vi "test TCX read (installed 71).vi"() -> ()   [LabVIEW 2011] (continued)
xmlns=\"http://www.garmin.com/xmlschemas/ActivityExtension/v2\"><Watts>67</Watts></TPX></Extensions></Trackpoint><Trackpoint><Time>2008-03-03T23:25:10Z</Time><Position><LatitudeDegrees>35.887956</LatitudeDegrees><LongitudeDegrees>-78.948106</LongitudeDegrees></Position><AltitudeMeters>75.120</AltitudeMeters><DistanceMeters>21918.861</DistanceMeters><Cadence>88</Cadence><Extensions><TPX xmlns=\"http://www.garmin.com/xmlschemas/ActivityExtension/v2\"><Watts>54</Watts></TPX></Extensions></Trackpoint><Trackpoint><Time>2008-03-03T23:25:11Z</Time><Position><LatitudeDegrees>35.888009</LatitudeDegrees><LongitudeDegrees>-78.948257</LongitudeDegrees></Position><AltitudeMeters>74.640</AltitudeMeters><DistanceMeters>21933.953</DistanceMeters><Cadence>89</Cadence><Extensions><TPX xmlns=\"http://www.garmin.com/xmlschemas/ActivityExtension/v2\"><Watts>47</Watts></TPX></Extensions></Trackpoint><Trackpoint><Time>2008-03-03T23:25:12Z</Time><Position><LatitudeDegrees>35.888052</LatitudeDegrees><LongitudeDegrees>-78.948414</LongitudeDegrees></Position><AltitudeMeters>72.717</AltitudeMeters><DistanceMeters>21948.695</DistanceMeters><Cadence>90</Cadence><Extensions><TPX xmlns=\"http://www.garmin.com/xmlschemas/ActivityExtension/v2\"><Watts>43</Watts></TPX></Extensions></Trackpoint><Trackpoint><Time>2008-03-03T23:25:13Z</Time><Position><LatitudeDegrees>35.888082</LatitudeDegrees><LongitudeDegrees>-78.948575</LongitudeDegrees></Position><AltitudeMeters>72.236</AltitudeMeters><DistanceMeters>21963.564</DistanceMeters><Cadence>89</Cadence><Extensions><TPX xmlns=\"http://www.garmin.com/xmlschemas/ActivityExtension/v2\"><Watts>44</Watts></TPX></Extensions></Trackpoint><Trackpoint><Time>2008-03-03T23:25:14Z</Time><Position><LatitudeDegrees>35.888095</LatitudeDegrees><LongitudeDegrees>-78.948737</LongitudeDegrees></Position><AltitudeMeters>72.236</AltitudeMeters><DistanceMeters>21978.184</DistanceMeters><Cadence>87</Cadence><Extensions><TPX xmlns=\"http://www.garmin.com/xmlschemas/ActivityExtension/v2\"><Watts>41</Watts></TPX></Extensions></Trackpoint><Trackpoint><Time>2008-03-03T23:25:15Z</Time><Position><LatitudeDegrees>35.888094</LatitudeDegrees><LongitudeDegrees>-78.948896</LongitudeDegrees></Position><AltitudeMeters>72.236</AltitudeMeters><DistanceMeters>21992.566</DistanceMeters><Cadence>87</Cadence><Extensions><TPX xmlns=\"http://www.garmin.com/xmlschemas/ActivityExtension/v2\"><Watts>41</Watts></TPX></Extensions></Trackpoint><Trackpoint><Time>2008-03-03T23:25:16Z</Time><Position><LatitudeDegrees>35.888082</LatitudeDegrees><LongitudeDegrees>-78.949051</LongitudeDegrees></Position><AltitudeMeters>71.755</AltitudeMeters><DistanceMeters>22006.510</DistanceMeters><Cadence>0</Cadence></Trackpoint><Trackpoint><Time>2008-03-03T23:25:17Z</Time><Position><LatitudeDegrees>35.888058</LatitudeDegrees><LongitudeDegrees>-78.949199</LongitudeDegrees></Position><AltitudeMeters>71.275</AltitudeMeters><DistanceMeters>22020.152</DistanceMeters><Cadence>0</Cadence></Trackpoint><Trackpoint><Time>2008-03-03T23:25:18Z</Time><Position><LatitudeDegrees>35.888029</LatitudeDegrees><LongitudeDegrees>-78.949342</LongitudeDegrees></Position><AltitudeMeters>71.275</AltitudeMeters><DistanceMeters>22033.473</DistanceMeters><Cadence>17</Cadence></Trackpoint><Trackpoint><Time>2008-03-03T23:25:19Z</Time><Position><LatitudeDegrees>35.888005</LatitudeDegrees><LongitudeDegrees>-78.949482</LongitudeDegrees></Position><AltitudeMeters>71.275</AltitudeMeters><DistanceMeters>22046.338</DistanceMeters><Cadence>33</Cadence></Trackpoint><Trackpoint><Time>2008-03-03T23:25:20Z</Time><Position><LatitudeDegrees>35.888007</LatitudeDegrees><LongitudeDegrees>-78.949623</LongitudeDegrees></Position><AltitudeMeters>70.794</AltitudeMeters><DistanceMeters>22058.844</DistanceMeters><Cadence>33</Cadence></Trackpoint><Trackpoint><Time>2008-03-03T23:25:21Z</Time><Position><LatitudeDegrees>35.888061</LatitudeDegrees><LongitudeDegrees>-78.949736</LongitudeDegrees></Position><AltitudeMeters>70.794</AltitudeMeters><DistanceMeters>22070.695</DistanceMeters><Cadence>0</Cadence></Trackpoint><Trackpoint><Time>2008-03-03T23:25:22Z</Time><Position><LatitudeDegrees>35.888146</LatitudeDegrees><LongitudeDegrees>-78.949802</LongitudeDegrees></Position><AltitudeMeters>70.794</AltitudeMeters><DistanceMeters>22081.836</DistanceMeters><Cadence>89</Cadence><Extensions><TPX xmlns=\"http://www.garmin.com/xmlschemas/ActivityExtension/v2\"><Watts>68</Watts></TPX></Extensions></Trackpoint><Trackpoint><Time>2008-03-03T23:25:23Z</Time><Position><LatitudeDegrees>35.888236</LatitudeDegrees><LongitudeDegrees>-78.949853</LongitudeDegrees></Position><AltitudeMeters>70.794</AltitudeMeters><DistanceMeters>22092.775</DistanceMeters><Cadence>89</Cadence><Extensions><TPX xmlns=\"http://www.garmin.com/xmlschemas/ActivityExtension/v2\"><Watts>73</Watts></TPX></Extensions></Trackpoint><Trackpoint><Time>2008-03-03T23:25:24Z</Time><Position><LatitudeDegrees>35.888330</LatitudeDegrees><LongitudeDegrees>-78.949892</LongitudeDegrees></Position><AltitudeMeters>70.794</AltitudeMeters><DistanceMeters>22103.824</DistanceMeters><Cadence>80</Cadence><Extensions><TPX xmlns=\"http://www.garmin.com/xmlschemas/ActivityExtension/v2\"><Watts>113</Watts></TPX></Extensions></Trackpoint><Trackpoint><Time>2008-03-03T23:25:25Z</Time><Position><LatitudeDegrees>35.888423</LatitudeDegrees><LongitudeDegrees>-78.949920</LongitudeDegrees></Position><AltitudeMeters>70.794</AltitudeMeters><DistanceMeters>22114.348</DistanceMeters><Cadence>80</Cadence><Extensions><TPX xmlns=\"http://www.garmin.com/xmlschemas/ActivityExtension/v2\"><Watts>112</Watts></TPX></Extensions></Trackpoint><Trackpoint><Time>2008-03-03T23:25:26Z</Time><Position><LatitudeDegrees>35.888512</LatitudeDegrees><LongitudeDegrees>-78.949941</LongitudeDegrees></Position><AltitudeMeters>70.794</AltitudeMeters><DistanceMeters>22124.379</DistanceMeters><Cadence>82</Cadence><Extensions><TPX xmlns=\"http://www.garmin.com/xmlschemas/ActivityExtension/v2\"><Watts>127</Watts></TPX></Extensions></Trackpoint><Trackpoint><Time>2008-03-03T23:25:27Z</Time><Position><LatitudeDegrees>35.888597</LatitudeDegrees><LongitudeDegrees>-78.949963</LongitudeDegrees></Position><AltitudeMeters>70.313</AltitudeMeters><DistanceMeters>22134.072</DistanceMeters><Cadence>78</Cadence><Extensions><TPX xmlns=\"http://www.garmin.com/xmlschemas/ActivityExtension/v2\"><Watts>137</Watts></TPX></Extensions></Trackpoint><Trackpoint><Time>2008-03-03T23:25:28Z</Time><Position><LatitudeDegrees>35.888682</LatitudeDegrees><LongitudeDegrees>-78.949991</LongitudeDegrees></Position><AltitudeMeters>70.794</AltitudeMeters><DistanceMeters>22143.781</DistanceMeters><Cadence>78</Cadence><Extensions><TPX xmlns=\"http://www.garmin.com/xmlschemas/ActivityExtension/v2\"><Watts>234</Watts></TPX></Extensions></Trackpoint><Trackpoint><Time>2008-03-03T23:25:29Z</Time><Position><LatitudeDegrees>35.888765</LatitudeDegrees><LongitudeDegrees>-78.950025</LongitudeDegrees></Position><AltitudeMeters>70.794</AltitudeMeters><DistanceMeters>22153.506</DistanceMeters><Cadence>78</Cadence><Extensions><TPX xmlns=\"http://www.garmin.com/xmlschemas/ActivityExtension/v2\"><Watts>358</Watts></TPX></Extensions></Trackpoint><Trackpoint><Time>2008-03-03T23:25:30Z</Time><Position><LatitudeDegrees>35.888845</LatitudeDegrees><LongitudeDegrees>-78.950066</LongitudeDegrees></Position><AltitudeMeters>71.275</AltitudeMeters><DistanceMeters>22163.023</DistanceMeters><Cadence>78</Cadence><Extensions><TPX xmlns=\"http://www.garmin.com/xmlschemas/ActivityExtension/v2\"><Watts>358</Watts></TPX></Extensions></Trackpoint><Trackpoint><Time>2008-03-03T23:25:31Z</Time><Position><LatitudeDegrees>35.888920</LatitudeDegrees><LongitudeDegrees>-78.950108</LongitudeDegrees></Position><AltitudeMeters>71.755</AltitudeMeters><DistanceMeters>22172.158</DistanceMeters><Cadence>73</Cadence><Extensions><TPX xmlns=\"http://www.garmin.com/xmlschemas/ActivityExtension/v2\"><Watts>561</Watts></TPX></Extensions></Trackpoint><Trackpoint><Time>2008-03-03T23:25:32Z</Time><Position><LatitudeDegrees>35.888993</LatitudeDegrees><LongitudeDegrees>-78.950147</LongitudeDegrees></Position><AltitudeMeters>72.717</AltitudeMeters><DistanceMeters>22181.043</DistanceMeters><Cadence>71</Cadence><Extensions><TPX xmlns=\"http://www.garmin.com/xmlschemas/ActivityExtension/v2\"><Watts>610</Watts></TPX></Extensions></Trackpoint><Trackpoint><Time>2008-03-03T23:25:33Z</Time><Position><LatitudeDegrees>35.889063</LatitudeDegrees><LongitudeDegrees>-78.950189</LongitudeDegrees></Position><AltitudeMeters>73.198</AltitudeMeters><DistanceMeters>22189.660</DistanceMeters><Cadence>71</Cadence><Extensions><TPX xmlns=\"http://www.garmin.com/xmlschemas/ActivityExtension/v2\"><Watts>609</Watts></TPX></Extensions></Trackpoint><Trackpoint><Time>2008-03-03T23:25:34Z</Time><Position><LatitudeDegrees>35.889129</LatitudeDegrees><LongitudeDegrees>-78.950236</LongitudeDegrees></Position><AltitudeMeters>74.159</AltitudeMeters><DistanceMeters>22198.082</DistanceMeters><Cadence>68</Cadence><Extensions><TPX xmlns=\"http://www.garmin.com/xmlschemas/ActivityExtension/v2\"><Watts>594</Watts></TPX></Extensions></Trackpoint><Trackpoint><Time>2008-03-03T23:25:35Z</Time><Position><LatitudeDegrees>35.889194</LatitudeDegrees><LongitudeDegrees>-78.950285</LongitudeDegrees></Position><AltitudeMeters>74.640</AltitudeMeters><DistanceMeters>22206.525</DistanceMeters><Cadence>67</Cadence><Extensions><TPX xmlns=\"http://www.garmin.com/xmlschemas/ActivityExtension/v2\"><Watts>574</Watts></TPX></Extensions></Trackpoint><Trackpoint><Time>2008-03-03T23:25:36Z</Time><Position><LatitudeDegrees>35.889252</LatitudeDegrees><LongitudeDegrees>-78.950341</LongitudeDegrees></Position><AltitudeMeters>74.640</AltitudeMeters><DistanceMeters>22214.654</DistanceMeters><Cadence>67</Cadence><Extensions><TPX xmlns=\"http://www.garmin.com/xmlschemas/ActivityExtension/v2\"><Watts>549</Watts></TPX></Extensions></Trackpoint><Trackpoint><Time>2008-03-03T23:25:37Z</Time><Position><LatitudeDegrees>35.889306</LatitudeDegrees><LongitudeDegrees>-78.950404</LongitudeDegrees></Position><AltitudeMeters>75.120</AltitudeMeters><DistanceMeters>22222.992</DistanceMeters><Cadence>67</Cadence><Extensions><TPX xmlns=\"http://www.garmin.com/xmlschemas/ActivityExtension/v2\"><Watts>534</Watts></TPX></Extensions></Trackpoint><Trackpoint><Time>2008-03-03T23:25:38Z</Time><Position><LatitudeDegrees>35.889357</LatitudeDegrees><LongitudeDegrees>-78.950472</LongitudeDegrees></Position><AltitudeMeters>75.601</AltitudeMeters><DistanceMeters>22231.277</DistanceMeters><Cadence>67</Cadence><Extensions><TPX xmlns=\"http://www.garmin.com/xmlschemas/ActivityExtension/v2\"><Watts>523</Watts></TPX></Extensions></Trackpoint><Trackpoint><Time>2008-03-03T23:25:39Z</Time><Position><LatitudeDegrees>35.889403</LatitudeDegrees><LongitudeDegrees>-78.950544</LongitudeDegrees></Position><AltitudeMeters>75.601</AltitudeMeters><DistanceMeters>22239.598</DistanceMeters><Cadence>69</Cadence><Extensions><TPX xmlns=\"http://www.garmin.com/xmlschemas/ActivityExtension/v2\"><Watts>356</Watts></TPX></Extensions></Trackpoint><Trackpoint><Time>2008-03-03T23:25:40Z</Time><Position><LatitudeDegrees>35.889447</LatitudeDegrees><LongitudeDegrees>-78.950625</LongitudeDegrees></Position><AltitudeMeters>76.562</AltitudeMeters><DistanceMeters>22248.361</DistanceMeters><Cadence>69</Cadence><Extensions><TPX xmlns=\"http://www.garmin.com/xmlschemas/ActivityExtension/v2\"><Watts>353</Watts></TPX></Extensions></Trackpoint><Trackpoint><Time>2008-03-03T23:25:41Z</Time><Position><LatitudeDegrees>35.889484</LatitudeDegrees><LongitudeDegrees>-78.950711</LongitudeDegrees></Position><AltitudeMeters>76.081</AltitudeMeters><DistanceMeters>22257.133</DistanceMeters><Cadence>71</Cadence><Extensions><TPX xmlns=\"http://www.garmin.com/xmlschemas/ActivityExtension/v2\"><Watts>275</Watts></TPX></Extensions></Trackpoint><Trackpoint><Time>2008-03-03T23:25:42Z</Time><Position><LatitudeDegrees>35.889518</LatitudeDegrees><LongitudeDegrees>-78.950802</LongitudeDegrees></Position><AltitudeMeters>75.601</AltitudeMeters><DistanceMeters>22266.189</DistanceMeters><Cadence>71</Cadence><Extensions><TPX xmlns=\"http://www.garmin.com/xmlschemas/ActivityExtension/v2\"><Watts>270</Watts></TPX></Extensions></Trackpoint><Trackpoint><Time>2008-03-03T23:25:43Z</Time><Position><LatitudeDegrees>35.889549</LatitudeDegrees><LongitudeDegrees>-78.950897</LongitudeDegrees></Position><AltitudeMeters>76.081</AltitudeMeters><DistanceMeters>22275.441</DistanceMeters><Cadence>77</Cadence><Extensions><TPX xmlns=\"http://www.garmin.com/xmlschemas/ActivityExtension/v2\"><Watts>84</Watts></TPX></Extensions></Trackpoint><Trackpoint><Time>2008-03-03T23:25:44Z</Time><Position><LatitudeDegrees>35.889575</LatitudeDegrees><LongitudeDegrees>-78.950998</LongitudeDegrees></Position><AltitudeMeters>75.601</AltitudeMeters><DistanceMeters>22285.012</DistanceMeters><Cadence>79</Cadence><Extensions><TPX xmlns=\"http://www.garmin.com/xmlschemas/ActivityExtension/v2\"><Watts>51</Watts></TPX></Extensions></Trackpoint><Trackpoint><Time>2008-03-03T23:25:45Z</Time><Position><LatitudeDegrees>35.889595</LatitudeDegrees><LongitudeDegrees>-78.951104</LongitudeDegrees></Position><AltitudeMeters>74.640</AltitudeMeters><DistanceMeters>22294.938</DistanceMeters><Cadence>79</Cadence><Extensions><TPX xmlns=\"http://www.garmin.com/xmlschemas/ActivityExtension/v2\"><Watts>51</Watts></TPX></Extensions></Trackpoint><Trackpoint><Time>2008-03-03T23:25:46Z</Time><Position><LatitudeDegrees>35.889610</LatitudeDegrees><LongitudeDegrees>-78.951218</LongitudeDegrees></Position><AltitudeMeters>74.159</AltitudeMeters><DistanceMeters>22305.377</DistanceMeters><Cadence>82</Cadence><Extensions><TPX xmlns=\"http://www.garmin.com/xmlschemas/ActivityExtension/v2\"><Watts>37</Watts></TPX></Extensions></Trackpoint><Trackpoint><Time>2008-03-03T23:25:47Z</Time><Position><LatitudeDegrees>35.889616</LatitudeDegrees><LongitudeDegrees>-78.951337</LongitudeDegrees></Position><AltitudeMeters>73.678</AltitudeMeters><DistanceMeters>22316.143</DistanceMeters><Cadence>82</Cadence><Extensions><TPX xmlns=\"http://www.garmin.com/xmlschemas/ActivityExtension/v2\"><Watts>37</Watts></TPX></Extensions></Trackpoint><Trackpoint><Time>2008-03-03T23:25:48Z</Time><Position><LatitudeDegrees>35.889598</LatitudeDegrees><LongitudeDegrees>-78.951455</LongitudeDegrees></Position><AltitudeMeters>73.198</AltitudeMeters><DistanceMeters>22326.912</DistanceMeters><Cadence>0</Cadence></Trackpoint><Trackpoint><Time>2008-03-03T23:25:49Z</Time><Position><LatitudeDegrees>35.889510</LatitudeDegrees><LongitudeDegrees>-78.951561</LongitudeDegrees></Position><AltitudeMeters>72.717</AltitudeMeters><DistanceMeters>22340.641</DistanceMeters><Cadence>0</Cadence></Trackpoint><Trackpoint><Time>2008-03-03T23:25:50Z</Time><Position><LatitudeDegrees>35.889400</LatitudeDegrees><LongitudeDegrees>-78.951620</LongitudeDegrees></Position><AltitudeMeters>72.717</AltitudeMeters><DistanceMeters>22353.893</DistanceMeters><Cadence>13</Cadence></Trackpoint><Trackpoint><Time>2008-03-03T23:25:51Z</Time><Position><LatitudeDegrees>35.889295</LatitudeDegrees><LongitudeDegrees>-78.951645</LongitudeDegrees></Position><AltitudeMeters>72.717</AltitudeMeters><DistanceMeters>22365.746</DistanceMeters><Cadence>85</Cadence><Extensions><TPX xmlns=\"http://www.garmin.com/xmlschemas/ActivityExtension/v2\"><Watts>34</Watts></TPX></Extensions></Trackpoint><Trackpoint><Time>2008-03-03T23:25:52Z</Time><Position><LatitudeDegrees>35.889198</LatitudeDegrees><LongitudeDegrees>-78.951661</LongitudeDegrees></Position><AltitudeMeters>71.755</AltitudeMeters><DistanceMeters>22376.627</DistanceMeters><Cadence>85</Cadence><Extensions><TPX xmlns=\"http://www.garmin.com/xmlschemas/ActivityExtension/v2\"><Watts>46</Watts></TPX></Extensions></Trackpoint><Trackpoint><Time>2008-03-03T23:25:53Z</Time><Position><LatitudeDegrees>35.889108</LatitudeDegrees><LongitudeDegrees>-78.951687</LongitudeDegrees></Position><AltitudeMeters>70.794</AltitudeMeters><DistanceMeters>22386.820</DistanceMeters><Cadence>84</Cadence><Extensions><TPX xmlns=\"http://www.garmin.com/xmlschemas/ActivityExtension/v2\"><Watts>46</Watts></TPX></Extensions></Trackpoint><Trackpoint><Time>2008-03-03T23:25:54Z</Time><Position><LatitudeDegrees>35.889030</LatitudeDegrees><LongitudeDegrees>-78.951733</LongitudeDegrees></Position><AltitudeMeters>71.275</AltitudeMeters><DistanceMeters>22396.348</DistanceMeters><Cadence>84</Cadence><Extensions><TPX xmlns=\"http://www.garmin.com/xmlschemas/ActivityExtension/v2\"><Watts>46</Watts></TPX></Extensions></Trackpoint><Trackpoint><Time>2008-03-03T23:25:55Z</Time><Position><LatitudeDegrees>35.888976</LatitudeDegrees><LongitudeDegrees>-78.951800</LongitudeDegrees></Position><AltitudeMeters>70.313</AltitudeMeters><DistanceMeters>22404.639</DistanceMeters><Cadence>0</Cadence></Trackpoint><Trackpoint><Time>2008-03-03T23:25:56Z</Time><Position><LatitudeDegrees>35.888968</LatitudeDegrees><LongitudeDegrees>-78.951871</LongitudeDegrees></Position><AltitudeMeters>70.313</AltitudeMeters><DistanceMeters>22411.021</DistanceMeters><Cadence>0</Cadence></Trackpoint><Trackpoint><Time>2008-03-03T23:25:57Z</Time><Position><LatitudeDegrees>35.888992</LatitudeDegrees><LongitudeDegrees>-78.951918</LongitudeDegrees></Position><AltitudeMeters>70.313</AltitudeMeters><DistanceMeters>22416.049</DistanceMeters><Cadence>0</Cadence></Trackpoint><Trackpoint><Time>2008-03-03T23:25:58Z</Time><Position><LatitudeDegrees>35.889021</LatitudeDegrees><LongitudeDegrees>-78.951943</LongitudeDegrees></Position><AltitudeMeters>70.313</AltitudeMeters><DistanceMeters>22420.010</DistanceMeters><Cadence>0</Cadence></Trackpoint><Trackpoint><Time>2008-03-03T23:25:59Z</Time><Position><LatitudeDegrees>35.889040</LatitudeDegrees><LongitudeDegrees>-78.951955</LongitudeDegrees></Position><AltitudeMeters>70.313</AltitudeMeters><DistanceMeters>22422.236</DistanceMeters><Cadence>11</Cadence></Trackpoint><Trackpoint><Time>2008-03-03T23:26:00Z</Time><Position><LatitudeDegrees>35.889049</LatitudeDegrees><LongitudeDegrees>-78.951956</LongitudeDegrees></Position><AltitudeMeters>70.313</AltitudeMeters><DistanceMeters>22422.754</DistanceMeters><Cadence>11</Cadence></Trackpoint><Trackpoint><Time>2008-03-03T23:26:01Z</Time><Position><LatitudeDegrees>35.889050</LatitudeDegrees><LongitudeDegrees>-78.951955</LongitudeDegrees></Position><AltitudeMeters>70.313</AltitudeMeters><DistanceMeters>22422.754</DistanceMeters><Cadence>0</Cadence></Trackpoint><Trackpoint><Time>2008-03-03T23:26:02Z</Time><Position><LatitudeDegrees>35.889053</LatitudeDegrees><LongitudeDegrees>-78.951954</LongitudeDegrees></Position><AltitudeMeters>70.794</AltitudeMeters><DistanceMeters>22422.754</DistanceMeters><Cadence>0</Cadence></Trackpoint><Trackpoint><Time>2008-03-03T23:26:03Z</Time><Position><LatitudeDegrees>35.889051</LatitudeDegrees><LongitudeDegrees>-78.951955</LongitudeDegrees></Position><AltitudeMeters>70.794</AltitudeMeters><DistanceMeters>22422.951</DistanceMeters><Cadence>0</Cadence></Trackpoint><Trackpoint><Time>2008-03-03T23:26:04Z</Time><Position><LatitudeDegrees>35.889052</LatitudeDegrees><LongitudeDegrees>-78.951955</LongitudeDegrees></Position><AltitudeMeters>70.794</AltitudeMeters><DistanceMeters>22422.951</DistanceMeters><Cadence>0</Cadence></Trackpoint><Trackpoint><Time>2008-03-03T23:26:05Z</Time><Position><LatitudeDegrees>35.889052</LatitudeDegrees><LongitudeDegrees>-78.951953</LongitudeDegrees></Position><AltitudeMeters>70.794</AltitudeMeters><DistanceMeters>22422.951</DistanceMeters><Cadence>0</Cadence></Trackpoint><Trackpoint><Time>2008-03-03T23:26:06Z</Time><Position><LatitudeDegrees>35.889053</LatitudeDegrees><LongitudeDegrees>-78.951953</LongitudeDegrees></Position><AltitudeMeters>70.794</AltitudeMeters><DistanceMeters>22422.951</DistanceMeters><Cadence>0</Cadence></Trackpoint><Trackpoint><Time>2008-03-03T23:26:07Z</Time><Position><LatitudeDegrees>35.889053</LatitudeDegrees><LongitudeDegrees>-78.951953</LongitudeDegrees></Position><AltitudeMeters>70.794</AltitudeMeters><DistanceMeters>22422.951</DistanceMeters><Cadence>0</Cadence></Trackpoint><Trackpoint><Time>2008-03-03T23:26:08Z</Time><Position><LatitudeDegrees>35.889054</LatitudeDegrees><LongitudeDegrees>-78.951953</LongitudeDegrees></Position><AltitudeMeters>70.794</AltitudeMeters><DistanceMeters>22422.951</DistanceMeters><Cadence>0</Cadence></Trackpoint><Trackpoint><Time>2008-03-03T23:26:09Z</Time><Position><LatitudeDegrees>35.889055</LatitudeDegrees><LongitudeDegrees>-78.951953</LongitudeDegrees></Position><AltitudeMeters>70.794</AltitudeMeters><DistanceMeters>22422.951</DistanceMeters></Trackpoint><Trackpoint><Time>2008-03-03T23:26:10Z</Time><Position><LatitudeDegrees>35.889055</LatitudeDegrees><LongitudeDegrees>-78.951952</LongitudeDegrees></Position><AltitudeMeters>71.275</AltitudeMeters><DistanceMeters>22422.951</DistanceMeters></Trackpoint><Trackpoint><Time>2008-03-03T23:26:11Z</Time><Position><LatitudeDegrees>35.889056</LatitudeDegrees><LongitudeDegrees>-78.951951</LongitudeDegrees></Position><AltitudeMeters>71.275</AltitudeMeters><DistanceMeters>22422.951</DistanceMeters></Trackpoint><Trackpoint><Time>2008-03-03T23:26:12Z</Time><Position><LatitudeDegrees>35.889056</LatitudeDegrees><LongitudeDegrees>-78.951949</LongitudeDegrees></Position><AltitudeMeters>71.275</AltitudeMeters><DistanceMeters>22422.951</DistanceMeters></Trackpoint><Trackpoint><Time>2008-03-03T23:26:13Z</Time><Position><LatitudeDegrees>35.889057</LatitudeDegrees><LongitudeDegrees>-78.951949</LongitudeDegrees></Position><AltitudeMeters>71.275</AltitudeMeters><DistanceMeters>22422.951</DistanceMeters></Trackpoint><Trackpoint><Time>2008-03-03T23:26:14Z</Time><Position><LatitudeDegrees>35.889057</LatitudeDegrees><LongitudeDegrees>-78.951948</LongitudeDegrees></Position><AltitudeMeters>71.275</AltitudeMeters><DistanceMeters>22422.951</DistanceMeters></Trackpoint><Trackpoint><Time>2008-03-03T23:26:15Z</Time><Position><LatitudeDegrees>35.889057</LatitudeDegrees><LongitudeDegrees>-78.951947</LongitudeDegrees></Position><AltitudeMeters>70.794</AltitudeMeters><DistanceMeters>22422.951</DistanceMeters></Trackpoint><Trackpoint><Time>2008-03-03T23:26:16Z</Time><Position><LatitudeDegrees>35.889058</LatitudeDegrees><LongitudeDegrees>-78.951946</LongitudeDegrees></Position><AltitudeMeters>70.794</AltitudeMeters><DistanceMeters>22422.951</DistanceMeters></Trackpoint><Trackpoint><Time>2008-03-03T23:26:17Z</Time><Position><LatitudeDegrees>35.889058</LatitudeDegrees><LongitudeDegrees>-78.951945</LongitudeDegrees></Position><AltitudeMeters>70.794</AltitudeMeters><DistanceMeters>22422.951</DistanceMeters></Trackpoint><Trackpoint><Time>2008-03-03T23:26:18Z</Time><Position><LatitudeDegrees>35.889058</LatitudeDegrees><LongitudeDegrees>-78.951944</LongitudeDegrees></Position><AltitudeMeters>70.794</AltitudeMeters><DistanceMeters>22422.951</DistanceMeters></Trackpoint><Trackpoint><Time>2008-03-03T23:26:19Z</Time></Trackpoint></Track></Lap><Creator xsi:type=\"Device_t\"><Name>EDGE705</Name><UnitId>3393620054</UnitId><ProductID>625</ProductID><Version><VersionMajor>2</VersionMajor><VersionMinor>1</VersionMinor><BuildMajor>0</BuildMajor><BuildMinor>0</BuildMinor></Version></Creator></Activity></Activities><Author xsi:type=\"Application_t\"><Name>EDGE705</Name><Build><Version><VersionMajor>2</VersionMajor><VersionMinor>1</VersionMinor><BuildMajor>0</BuildMajor><BuildMinor>0</BuildMinor></Version><Type>Release</Type></Build><LangID>EN</LangID><PartNumber>006-B0625-00</PartNumber></Author></TrainingCenterDatabase>"
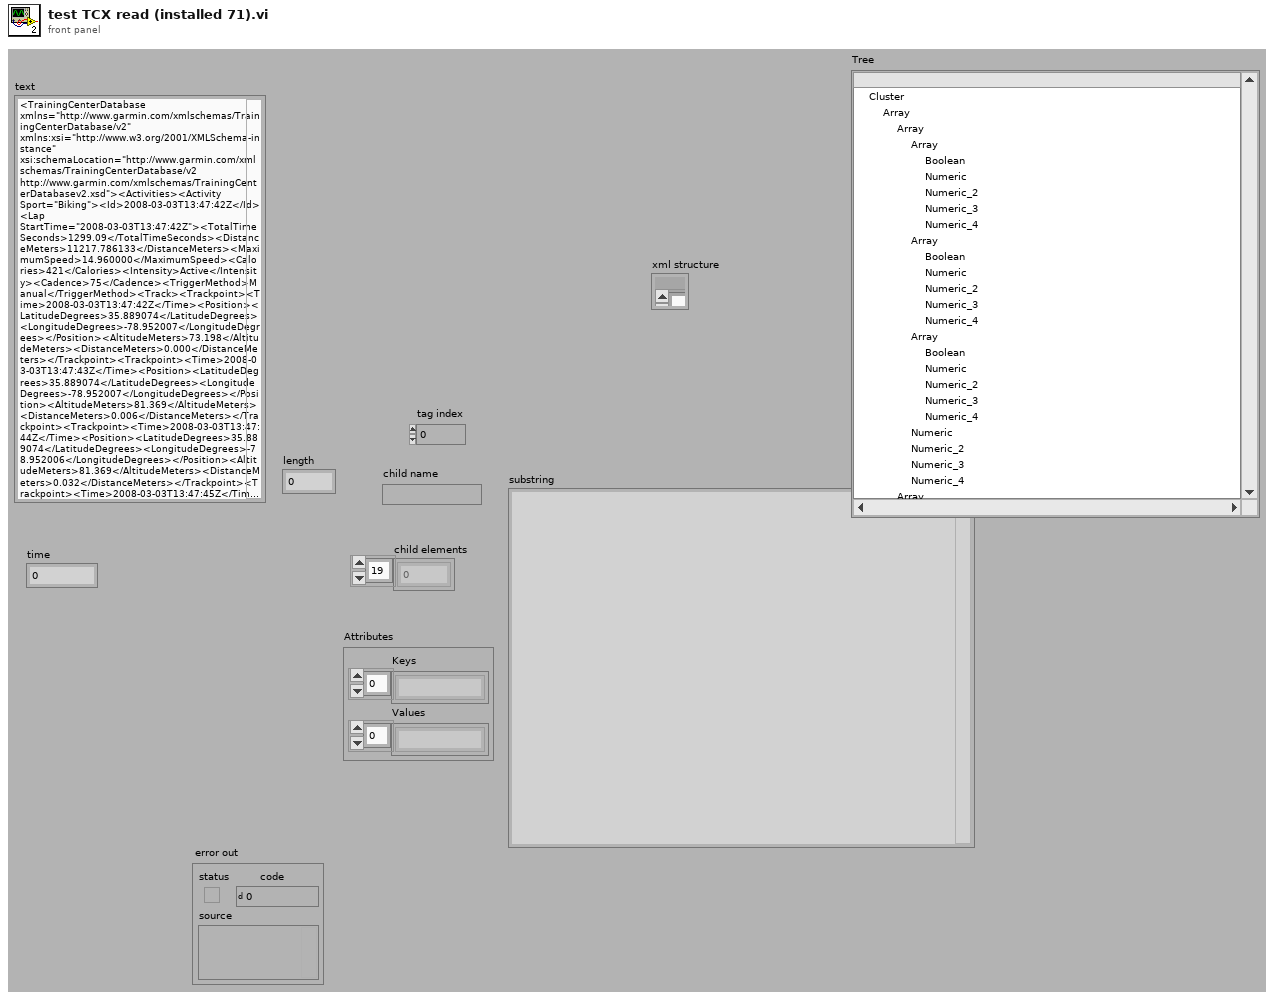
[diagram p1: front panel]
types:
  T1 = typedef "XML Structure - Cluster.ctl" = cluster{"tags":string[], "tag names":string[], "tag type":T2[], "offset":i32[], "close tag index":i32[], "xml":string, "Children":cluster{"children":i32[]}[], "parent index":i32[]}
  T2 = typedef "XML Tag Type - Enum.ctl" = enum16{"start tag", "empty tag", "end tag"}
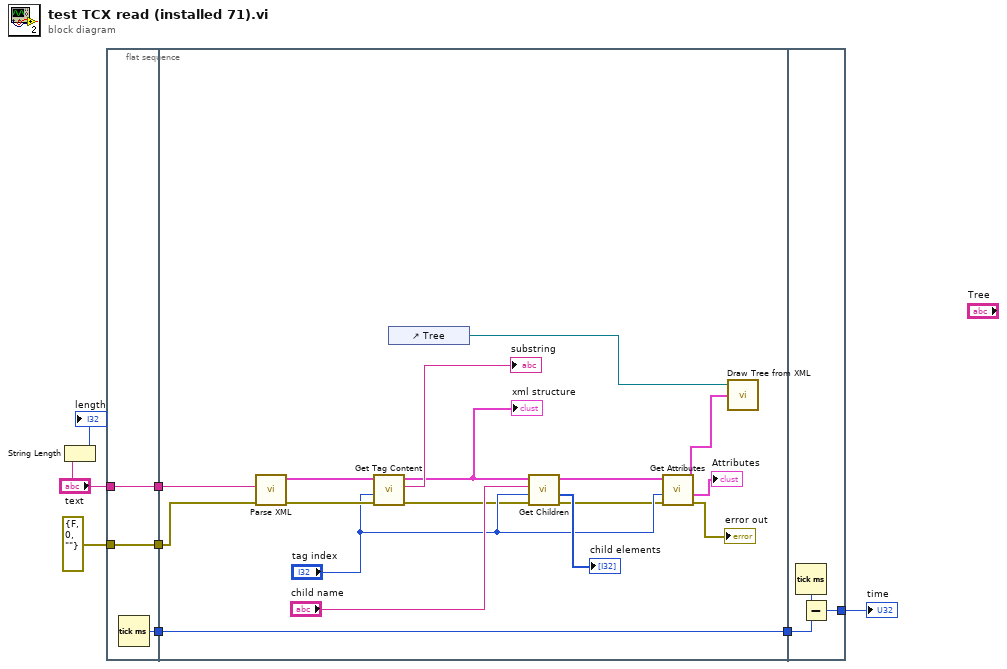
[diagram p0: block diagram]
diagram:
  n1 = String Length(string="text") -> (length=→"length":i32)
  n2 = flat-sequence {
    tunnel: "text" -> [w11]
    tunnel: [w11] -> w6
    tunnel: [w10] -> w5
    tunnel: [w9] -> w2
    tunnel: errorcluster {"status"=FALSE, "code"=0, "source"=""} ("error in (no error)") -> [w9]
    tunnel: [w28] -> w8
    tunnel: w6 -> [w18]
    tunnel: w5 -> [w28]
    tunnel: w2 -> [w17]
    tunnel: w8 -> [w30]
    tunnel: [w29] -> w7
    frame #0 {
      n3 = Tick Count (ms)() -> (millisecond timer value=w10:u32)
    }
    frame #1 {
      n4 = call "Parse XML.vi"("error in (no error)"=w17, "xml string"=w18) -> ("error out"=w25:errorcluster, "xml out"=w27:T1)  [unwired: 8 in]
      n5 = call "Get Tag Content.vi"("error in (no error)"=w25, "tag index"="tag index", "xml in"=w27) -> ("error out"=w15:errorcluster, "element content"=→"substring":string, "xml out"=w16:T1)  [unwired: 5 in, 1 out]
      "xml structure" <- w16
      n6 = control-ref of="Tree"() -> (w13:refnum<vi>)
      n7 = call "Get Children.vi"("error in (no error)"=w15, "tag index"="tag index", "child name (\"\": all children)"="child name", "xml structure in"=w16) -> ("error out"=w20:errorcluster, "child indices"=→"child elements":i32[], "xml structure out"=w22:T1)  [unwired: 4 in, 1 out]
      n8 = call "Get Attributes.vi"("error in (no error)"=w20, "tag index"="tag index", "xml structure in"=w22) -> ("error out"=→"error out":errorcluster, "Attributes"=→"Attributes":cluster{"Keys":string[], "Values":string[]}, "xml structure out"=w12:T1)  [unwired: 6 in]
      n9 = call "Draw Tree from XML.vi"("xml structure in"=w12, "reference"=w13) -> ()  [unwired: 1 in]
    }
    frame #2 {
      n10 = Tick Count (ms)() -> (millisecond timer value=w31:u32)
      n11 = Subtract(x=w31, y=w30) -> (x-y=w29:u32)
    }
  }
  "time" <- w7
